vi "Test LED Matrix.vi"() -> ()   [LabVIEW 2026]
uses:
  LED Matrix/LED Matrix/Display Configuration.ctl
  <vilib>/ActorFramework/Message Enqueuer/Message Enqueuer.lvclass/Message Enqueuer.ctl
  LED Matrix/Text/Text.lvclass
  home/pete/dev/labview-car/dev/LED Matrix/Content/Content.lvclass
  LED Matrix/LED Matrix Messages/Set Configuration Msg/Set Configuration Msg.lvclass/Set Configuration Msg.ctl
  <vilib>/ActorFramework/Message Enqueuer/Enqueue.vi
  LED Matrix/LED Matrix/LED Matrix.lvclass
  usr/local/natinst/LabVIEW-2026-64/vi.lib/ActorFramework/Actor/Actor.lvclass
  <vilib>/ActorFramework/Stop Msg/Stop Msg.lvclass
  usr/local/natinst/LabVIEW-2026-64/vi.lib/ActorFramework/Message/Message.lvclass
  LED Matrix/LED Matrix Messages/Set Configuration Msg/Set Configuration Msg.lvclass
  <vilib>/ActorFramework/Message Priority Queue/Priority Enqueue.vi
  home/pete/dev/labview-car/dev/LED Matrix/Text/Text.lvclass
  <vilib>/ActorFramework/Actor/Actor.lvclass
  CTI-Grove/Examples/Sourcecode/cti-drivers-lv-visa-simple/Examples/Driver/CTIPicoVISA.lvlib
panel:
  in  "LED Configuration":T1
  out "error out":errorcluster
  in  "stop":bool
  in  "VISA resource name":refnum<visa-resource-name>
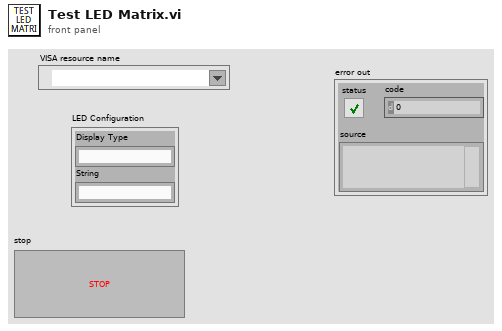
[diagram p1: front panel]
types:
  T1 = typedef "LED Matrix.lvlib/LED Matrix.lvclass/Display Configuration.ctl" = cluster{"Display Type":string, "String":string}
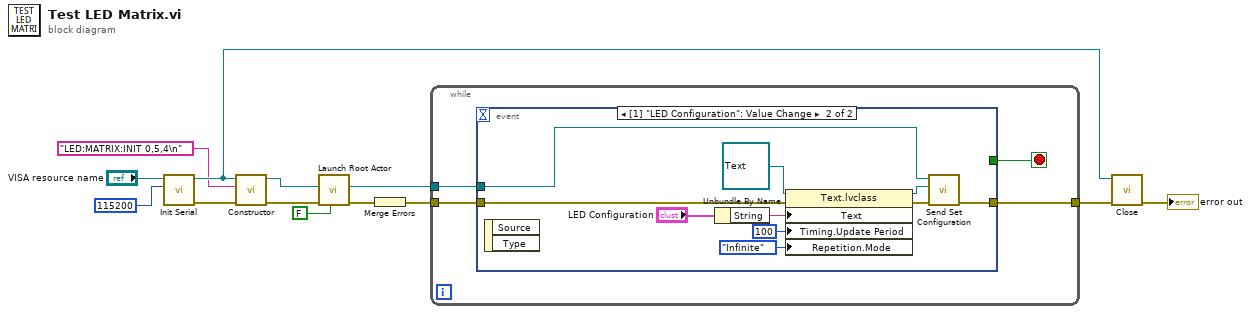
[diagram p0: block diagram]
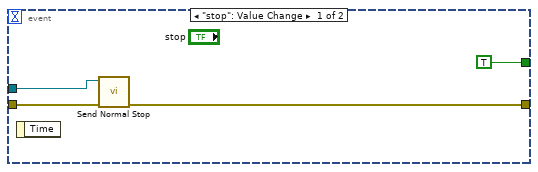
[diagram p2: hidden frame]
diagram:
  n1 = call "Init Serial.vi"("Baud (115200)"=u32 115200, "VISA resource name in"="VISA resource name") -> ("error out"=w10:errorcluster, "VISA resource name Out"=w5:refnum<visa-resource-name>)  [unwired: 7 in, 1 out]
  n2 = call "Constructor.vi"("error in (no error)"=w10, "Init Command"="LED:MATRIX:INIT 0,5,4\n" ("write buffer"), "VISA resource name"=w5) -> ("error out"=w3:errorcluster, "LED Matrix out"=w4:refnum<class "LED Matrix.lvclass">)  [unwired: 7 in]
  n3 = call <vilib>:"Launch Root Actor.vi"("Open Actor Core front panel? (F)"=FALSE, "error in (no error)"=w3, "Actor"=w4) -> ("error out"=w9:errorcluster, "Actor's Enqueuer"=w13:refnum<class "Message Enqueuer.lvclass">)  [unwired: 7 in]
  n4 = Merge Errors(w9) -> (w8:errorcluster)
  n5 = while {
    tunnel: w13 -> [w17]
    tunnel: [w15] -> w7
    tunnel: w8 -> [w14]
    stop <- w16 stop-if-true
    n6 = event shown="[1] \"LED Configuration\": Value Change" {
      selector: _ -> [_ _]
      dyn-events: _ -> [_ _]
      timeout: _ -> [_ _]
      tunnel: w17 -> [w21 w31]
      tunnel: [w20 w29] -> w15
      tunnel: [TRUE _] -> w16
      tunnel: w14 -> [w18 w30]
      event "stop": Value Change {
        n7 = event-data() -> ()  [unwired: 1 in, 1 out]
        n8 = call <vilib>:"Send Normal Stop.vi"("error in (no error)"=w18, "Message Enqueuer"=w21) -> ("error out"=w20:errorcluster)  [unwired: 9 in]
      }
      event Value Change {
        n9 = event-data() -> ()  [unwired: 1 in, 2 out]
        n10 = Unbundle By Name("LED Configuration") -> ("String"=w25:string)
        n11 = property class="Text.lvclass"(reference=refnum<class "Text.lvclass"> refnum ("LED Matrix.lvlib:Text.lvclass"), error in=w30, "Text"=w25, "Timing.Update Period"=100 ("Update Period"), "Repetition.Mode"=enum16{"Once", "Count", "Infinite"}."Infinite" ("Mode")) -> (reference out=w24:refnum<class "Text.lvclass">, error out=w28:errorcluster)
        n12 = call "Send Set Configuration.vi"("error in (no error)"=w28, "Content"=w24, "Message Enqueuer"=w31) -> ("error out"=w29:errorcluster)  [unwired: 7 in, 1 out]
      }
    }
  }
  n13 = call "Close.vi"("error in (no error)"=w7, "VISA resource name in"=w5) -> ("error out"=→"error out":errorcluster)  [unwired: 9 in]
